vi "Acquisition Message Loop.vi"(5 "UI Refs":T1, 8 "error in (no error)":errorcluster, 9 "Data Queue":refnum<queue>, 10 "Data Notifier":refnum<notifier>, 11 "Message Queues":T2) -> (0 "error out":errorcluster)   [LabVIEW 2018, in "Acquisition.lvlib"]
doc: "Message loop for handling messages pertaining to the acquisition of data from the hardware."
uses:
  Acquisition.lvlib
  support/Message Queue/All Message Queues.ctl
  support/Message Queue/Message Cluster.ctl
  controls/UI Data.ctl
  Hardware Configuration.ctl
  Acquisition State.ctl
  support/Message Queue/Enqueue Message (Single).vi
  <vilib>/Utility/error.llb/Error Cluster From Error Code.vi
  <vilib>/ErrorRing/Error Ring.xnode
  support/Message Queue/Message Queue.lvlib
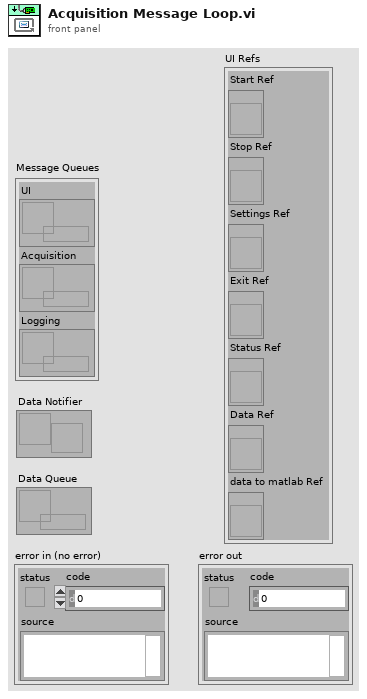
[diagram p1: front panel]
types:
  T1 = typedef "UI Data.ctl" = cluster{"Start Ref":refnum<vi>, "Stop Ref":refnum<vi>, "Settings Ref":refnum<vi>, "Exit Ref":refnum<vi>, "Status Ref":refnum<vi>, "Data Ref":refnum<vi>, "data to matlab Ref":refnum<vi>}
  T2 = typedef "Message Queue.lvlib/All Message Queues.ctl" = cluster{"UI":refnum<queue>, "Acquisition":refnum<queue>, "Logging":refnum<queue>}
  T3 = typedef "Acquisition.lvlib/Hardware Configuration.ctl" = cluster{"DAQmx Channel 1":tag, "DAQmx Channel 2":tag, "DAQmx Channel 3":tag, "Channel 1 Name":string, "Channel 2 Name":string, "Channel 3 Name":string, "Input Config Channel 1":i32, "Input Config Channel 2":i32, "Input Config Channel 3":i32, "Offset Channel 1":dbl, "Offset Channel 2":dbl, "Offset Channel 3":dbl, "Scale Channel 1":dbl, "Scale Channel 2":dbl, "Scale Channel 3":dbl, "Sample time":u32, "Samples per second":dbl, "Sample mode":u16, "Samples per channel":i32, "DAQmx AI Task":refnum<k21>, "DAQmx Channel 4":tag, "Channel 3 Name 2":string, "Input Config Channel 4":i32, "Offset Channel 4":dbl, "Scale Channel 4":dbl}
  T4 = typedef "Acquisition.lvlib/Acquisition State.ctl" = enum16{"Idle", "Acquiring"}
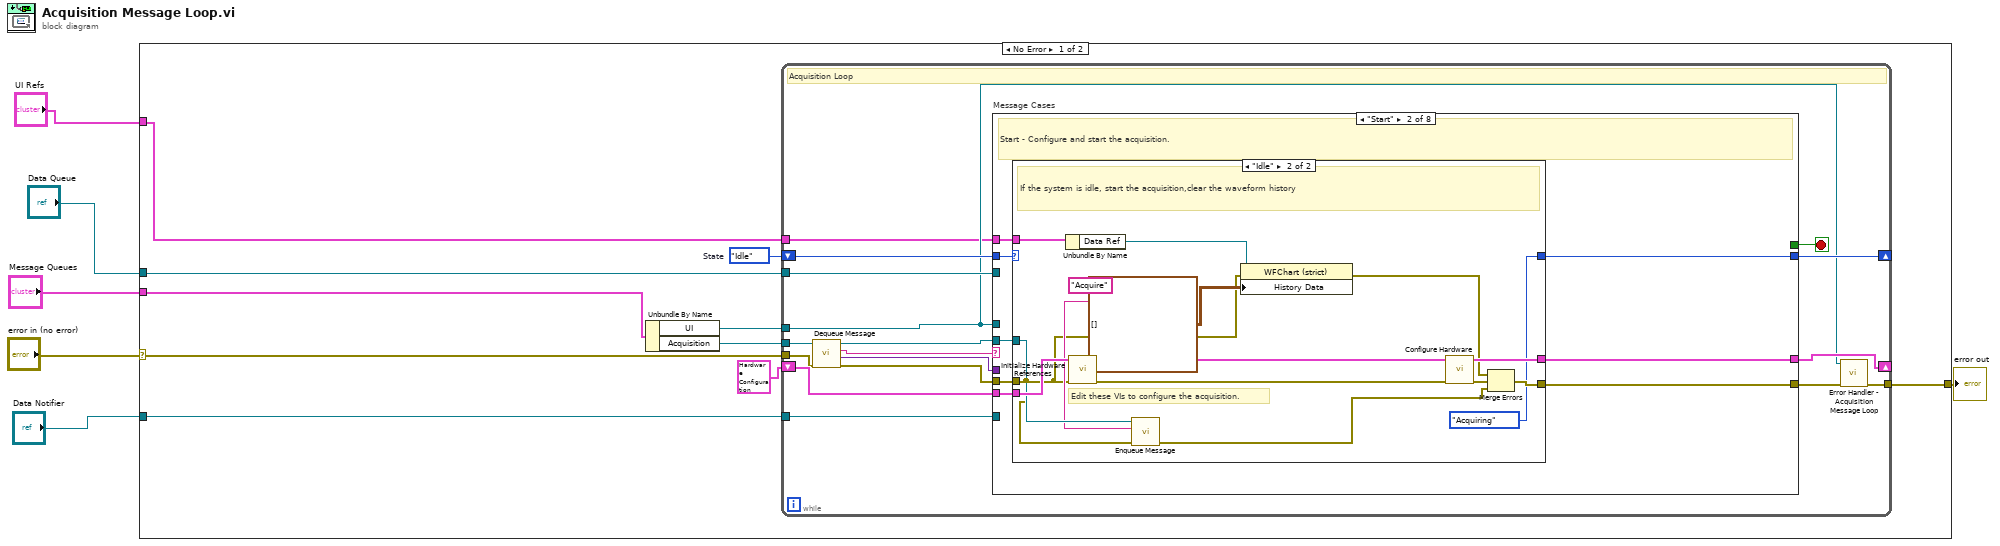
[diagram p0: block diagram]
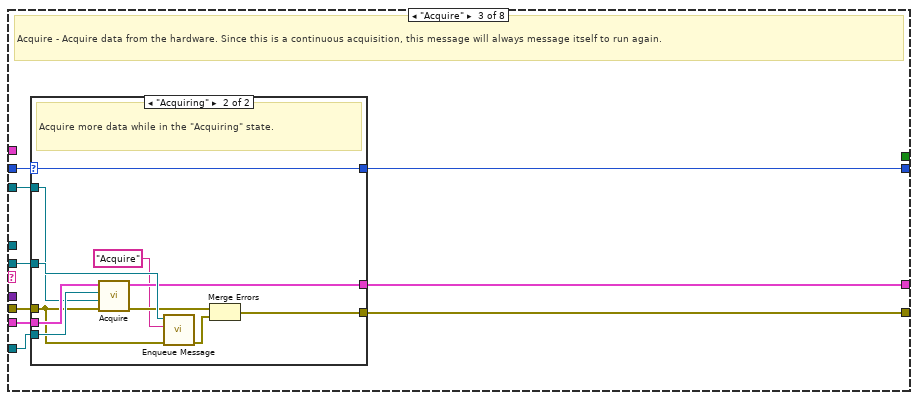
[diagram p4: hidden frame]
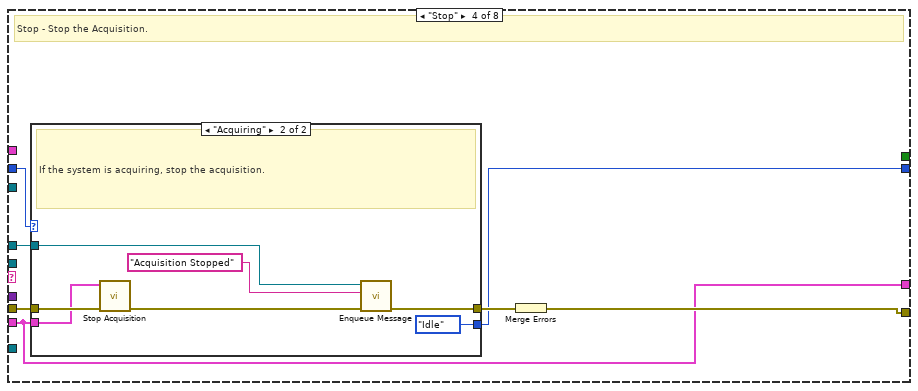
[diagram p6: hidden frame]
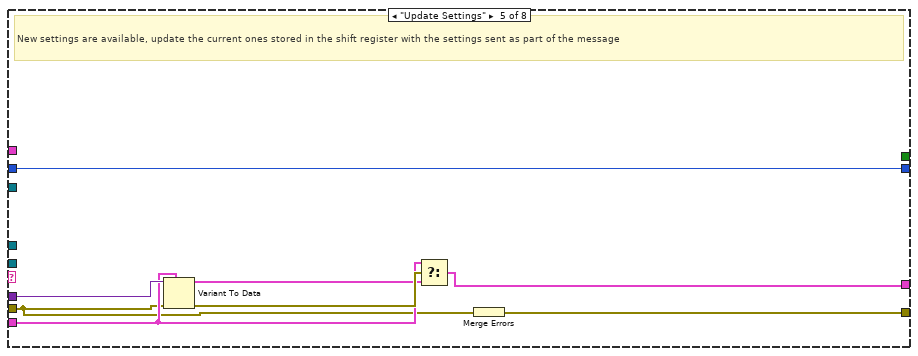
[diagram p8: hidden frame]
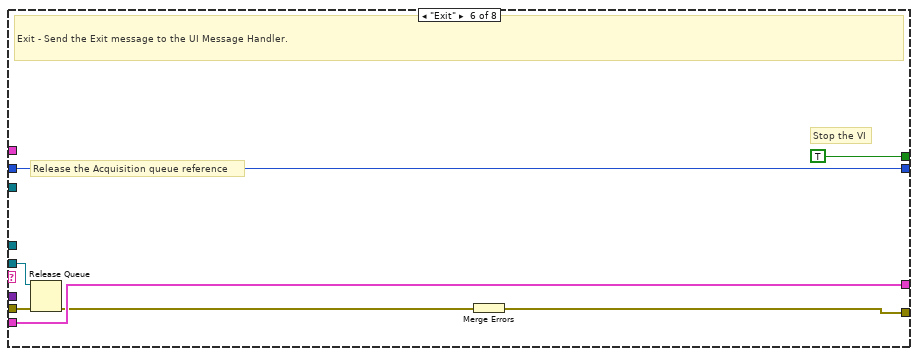
[diagram p9: hidden frame]
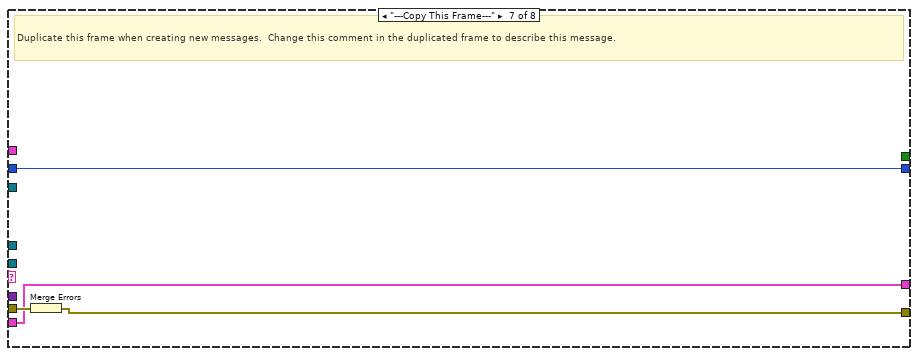
[diagram p10: hidden frame]
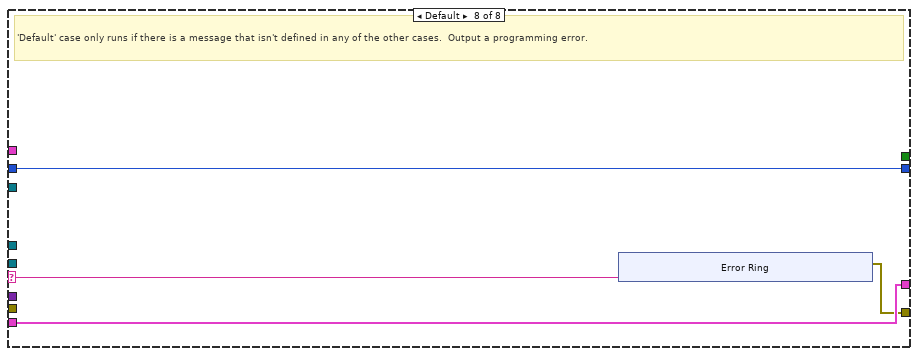
[diagram p11: hidden frame]
diagram:
  n1 = case shown="No Error" "error in (no error)" {
    selector: "error in (no error)" -> [w12 w132]
    tunnel: "Message Queues" -> [w16 _]
    tunnel: [w14 w132] -> w5
    tunnel: "Data Notifier" -> [w10 _]
    tunnel: "Data Queue" -> [w9 _]
    tunnel: "UI Refs" -> [w7 _]
    frame No Error {
      w8 = Acquisition_State."Idle"  # State
      n2 = Unbundle By Name(w16) -> ("UI"=w11:refnum<queue>, "Acquisition"=w15:refnum<queue>)
      n3 = while {
        tunnel: w15 -> [w26]
        shift-right: [w32] -> _
        shift-left: T3 {"DAQmx Channel 1"="", "DAQmx Channel 2"="", "DAQmx Channel 3"="", "Channel 1 Name"="Battery Voltage", "Channel 2 Name"="Battery Current", "Channel 3 Name"="Brake torque", "Input Config Channel 1"=-1, "Input Config Channel 2"=-1, "Input Config Channel 3"=-1, "Offset Channel 1"=0.0, "Offset Channel 2"=0.0, "Offset Channel 3"=0.0, "Scale Channel 1"=0.0, "Scale Channel 2"=0.0, "Scale Channel 3"=0.0, "Sample time"=50, "Samples per second"=1000.0, "Sample mode"=0, "Samples per channel"=0, "DAQmx AI Task"="", "DAQmx Channel 4"="", "Channel 3 Name 2"="", "Input Config Channel 4"=-1, "Offset Channel 4"=0.0, "Scale Channel 4"=0.0} ("Data Cluster") -> [w33]
        tunnel: w11 -> [w18]
        tunnel: w10 -> [w25]
        tunnel: w9 -> [w24]
        shift-right: [w22] -> _
        shift-left: w8 -> [w23]
        tunnel: w12 -> [w30]
        tunnel: [w21] -> w14
        tunnel: w7 -> [w17]
        stop <- w31 stop-if-true
        # "Acquisition Loop"
        n4 = call "Dequeue Message.vi"("error in (no error)"=w30, "Message Queue"=w26) -> ("error out"=w29:errorcluster, "Message Data"=w27:variant, "Message"=w28:string, "dup Message Queue"=w19:refnum<queue>)  [unwired: 6 in]
        n5 = case "Message Cases" shown="\"Start\"" w28 {
          selector: w28 -> [_ _ _ _ _ _ _ w121]
          tunnel: w19 -> [_ w41 w70 _ _ w111 _ _]
          tunnel: w29 -> [w36 w42 w69 w91 w103 w113 w120 _]
          tunnel: [w36 w44 w71 w92 w109 w115 w118 w122] -> w20
          tunnel: w33 -> [w35 w43 w67 w89 w105 w114 w119 w124]
          tunnel: [w35 w40 w68 w89 w104 w114 w119 w124] -> w32
          tunnel: [_ _ _ _ _ TRUE _ _] -> w31
          tunnel: w27 -> [_ _ _ _ w108 _ _ _]
          tunnel: w18 -> [_ _ _ w86 _ _ _ _]
          tunnel: w25 -> [_ _ w66 _ _ _ _ _]
          tunnel: w24 -> [_ _ w65 _ _ _ _ _]
          tunnel: w23 -> [w34 w38 w63 w88 w102 w110 w117 w123]
          tunnel: [w34 w39 w64 w87 w102 w110 w117 w123] -> w22
          tunnel: w17 -> [_ w37 _ _ _ _ _ _]
          frame "Initialize" {
            # "Initialize  - Initialize is currently a no-op.  The hardware initialization takes place in the 'Start' message."
          }
          frame "Start" {
            # "Start - Configure and start the acquisition."
            n6 = case shown="\"Idle\"" w38 {
              selector: w38 -> [w45 _]
              tunnel: [w46 w62] -> w44
              tunnel: w43 -> [w47 w61]
              tunnel: w42 -> [w46 w50]
              tunnel: w41 -> [_ w59]
              tunnel: [w47 w56] -> w40
              tunnel: [w45 Acquisition_State."Acquiring" ("Acquisition State")] -> w39
              tunnel: w37 -> [_ w48]
              frame "Acquiring" {
                # "The system is already acquiring. Ignore the \"Start\" message."
              }
              frame "Idle" {
                # "Edit these VIs to configure the acquisition."
                # "If the system is idle, start the acquisition,clear the waveform history"
                n7 = Unbundle By Name(w48) -> ("Data Ref"=w52:refnum<vi>)
                n8 = call "Initialize Hardware References.vi"("error in (no error)"=w50, "Hardware Resources in"=w61) -> ("error out"=w58:errorcluster, "Hardware Resources out"=w53:T3)  [unwired: 8 in]
                n9 = call-poly "Enqueue Message.vi"("error in (no error)"=w50, "Message"="Acquire", "Message Queue"=w59) -> ("error out"=w60:errorcluster)  [unwired: 7 in, 1 out]
                n10 = property class="WFChart (strict)"(reference=w52, error in=w50, "History Data"=waveform(dbl)[][] []) -> (error out=w49:errorcluster)  [unwired: 1 out]
                n11 = call "Configure Hardware.vi"("error in (no error)"=w58, "Hardware Resources in"=w53) -> ("error out"=w57:errorcluster, "Hardware Resources out"=w56:T3)  [unwired: 8 in]
                n12 = Merge Errors(w49, w57, w60) -> (w62:errorcluster)
              }
            }
          }
          frame "Acquire" {
            # "Acquire - Acquire data from the hardware. Since this is a continuous acquisition, this message will always message itself to run again."
            n13 = case shown="\"Acquiring\"" w63 {
              selector: w63 -> [w72 w76]
              tunnel: [w73 w85] -> w71
              tunnel: w70 -> [_ w83]
              tunnel: w69 -> [w73 w75]
              tunnel: [w74 w81] -> w68
              tunnel: w67 -> [w74 w80]
              tunnel: w66 -> [_ w78]
              tunnel: w65 -> [_ w77]
              tunnel: [w72 w76] -> w64
              frame "Idle" {
                # "Ignore \"Acquire\" messages when the acquisition is idle."
              }
              frame "Acquiring" {
                # "Acquire more data while in the \"Acquiring\" state."
                n14 = call "Acquire.vi"("error in (no error)"=w75, "Data Queue"=w77, "Data Notifier"=w78, "Hardware Resources in"=w80) -> ("error out"=w82:errorcluster, "Hardware Resources out"=w81:T3)  [unwired: 6 in]
                n15 = call-poly "Enqueue Message.vi"("error in (no error)"=w75, "Message"="Acquire", "Message Queue"=w83) -> ("error out"=w84:errorcluster)  [unwired: 7 in, 1 out]
                n16 = Merge Errors(w82, w84) -> (w85:errorcluster)
              }
            }
          }
          frame "Stop" {
            # "Stop - Stop the Acquisition."
            n17 = case shown="\"Acquiring\"" w88 {
              selector: w88 -> [w93 _]
              tunnel: w91 -> [w94 w101]
              tunnel: [w94 w97] -> w90
              tunnel: w89 -> [_ w99]
              tunnel: [w93 Acquisition_State."Idle" ("State")] -> w87
              tunnel: w86 -> [_ w96]
              frame "Idle" {
                # "The system is already idle. Ignore the \"Stop\" message."
              }
              frame "Acquiring" {
                # "If the system is acquiring, stop the acquisition."
                n18 = call "Stop Acquisition.vi"("error in (no error)"=w101, "Hardware Resources in"=w99) -> ("error out"=w100:errorcluster)  [unwired: 9 in]
                n19 = call-poly "Enqueue Message.vi"("error in (no error)"=w100, "Message"="Acquisition Stopped", "Message Queue"=w96) -> ("error out"=w97:errorcluster)  [unwired: 7 in, 1 out]
              }
            }
            n20 = Merge Errors(w90) -> (w92:errorcluster)
          }
          frame "Update Settings" {
            # "New settings are available, update the current ones stored in the shift register with the settings sent as part of the message"
            n21 = Variant To Data(error in=w103, type=w105, Variant=w108) -> (data=w106:T3, error out=w107:errorcluster)
            n22 = Select(t=w105, s=w107, f=w106) -> (s? t:f=w104:T3)
            n23 = Merge Errors(w103) -> (w109:errorcluster)
          }
          frame "Exit" {
            # "Release the Acquisition queue reference"
            # "Stop the VI"
            # "Exit - Send the Exit message to the UI Message Handler."
            n24 = Release Queue(queue=w111, error in (no error)=w113) -> (error out=w112:errorcluster)  [unwired: 1 in, 2 out]
            n25 = Merge Errors(w112) -> (w115:errorcluster)
          }
          frame "---Copy This Frame---" {
            # "Duplicate this frame when creating new messages.  Change this comment in the duplicated frame to describe this message."
            n26 = Merge Errors(w120) -> (w118:errorcluster)
          }
          frame Default {
            # "'Default' case only runs if there is a message that isn't defined in any of the other cases.  Output a programming error."
            n27 = xnode "Error Ring"("parameter 0"=w121) -> ("error out"=w122:errorcluster)
          }
        }
        n28 = call "Error Handler - Acquisition Message Loop.vi"("error in (no error)"=w20, "Message Queue"=w18) -> ("dup error in"=w21:errorcluster)  [unwired: 8 in, 1 out]
      }
    }
    frame Error {
    }
  }
  "error out" <- w5
